vi "Test Coffee Shop Add Cashier.vi"(8 "error in (no error)":errorcluster, 11 "Coffee Shop Test In":refnum<class "Coffee Shop Test.lvclass">) -> (0 "error out":errorcluster, 3 "Coffee Shop Test Out":refnum<class "Coffee Shop Test.lvclass">)   [LabVIEW 2020, in "Coffee Shop Test.lvclass"]
uses:
  Coffee Shop Test.lvclass
  Coffee Shop/Coffee Shop.lvclass
  <vilib>/Asteme/Triarc Framework/Process/Process.lvclass
  <vilib>/Asteme/LUnit/Test Case.lvclass
  C:/Program Files (x86)/National Instruments/LabVIEW 2020/vi.lib/Asteme/Triarc Framework/Application/Application.lvclass
  C:/Program Files (x86)/National Instruments/LabVIEW 2020/vi.lib/Asteme/Triarc Framework/Process/Process.lvclass
  C:/Program Files (x86)/National Instruments/LabVIEW 2020/vi.lib/Asteme/Triarc Framework/Base/Base.lvclass
  C:/Program Files (x86)/National Instruments/LabVIEW 2020/vi.lib/Asteme/Triarc Framework/Error Handler Interface/Error Handler Interface.lvclass
  C:/Program Files (x86)/National Instruments/LabVIEW 2020/vi.lib/Asteme/Triarc Framework/Logging/Logging.lvclass
  C:/Users/anton/Documents/GitHub/Triarc-Examples/Coffee Shop/Coffee Shop/Coffee Shop.lvclass
  <vilib>/Asteme/Triarc Framework/Application/Application.lvclass
  C:/Program Files (x86)/National Instruments/LabVIEW 2020/vi.lib/Asteme/Triarc Framework Test Suite/Application Test/Application Test.lvclass
  C:/Program Files (x86)/National Instruments/LabVIEW 2020/vi.lib/Asteme/Triarc Framework Test Suite/Process Test/Process Test.lvclass
  C:/Program Files (x86)/National Instruments/LabVIEW 2020/vi.lib/Asteme/Triarc Framework Test Suite/Base Class Test/Base Test.lvclass
  C:/Program Files (x86)/National Instruments/LabVIEW 2020/vi.lib/Asteme/LUnit/Test Case.lvclass
  C:/Users/anton/Documents/GitHub/Triarc-Examples/Coffee Shop/Coffee Shop Test/Coffee Shop Test.lvclass
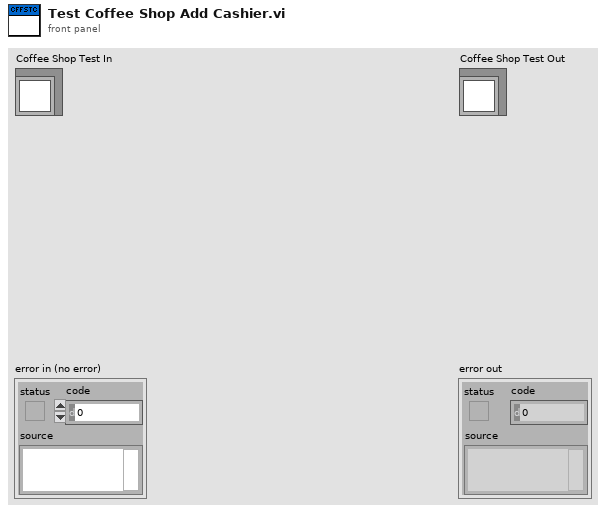
[diagram p1: front panel]
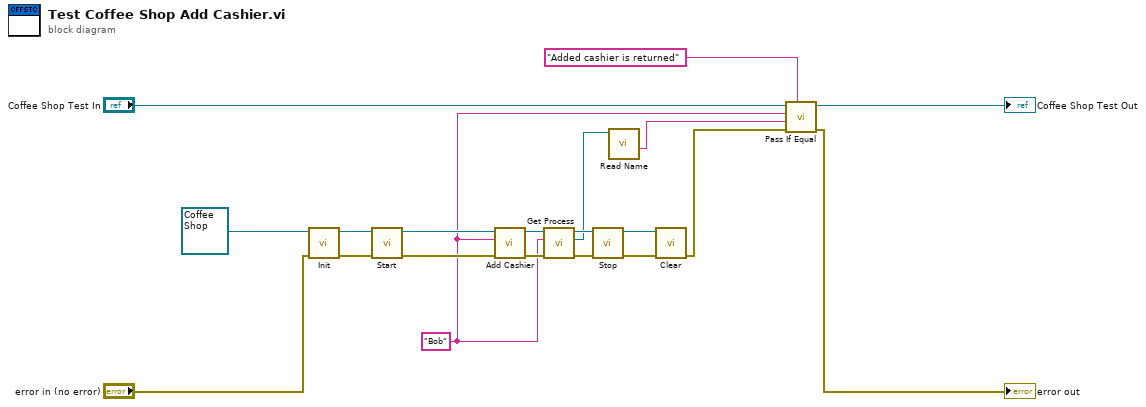
[diagram p0: block diagram]
diagram:
  w3 = "Bob" ("Name")
  n1 = call-dynamic "Init.vi"("error in (no error)"="error in (no error)", "Process In"=refnum<class "Coffee Shop.lvclass"> refnum ("Coffee Shop.lvclass")) -> ("error out"=w18:errorcluster, "Process Out"=w19:refnum<class "Coffee Shop.lvclass">)  [unwired: 8 in]
  n2 = call <vilib>:"Start.vi"("error in (no error)"=w18, "Process In"=w19) -> ("error out"=w13:errorcluster, "Process Out"=w12:refnum<class "Coffee Shop.lvclass">)  [unwired: 8 in]
  n3 = call "Add Cashier.vi"("error in (no error)"=w13, "Name"=w3, "Coffee Shop in"=w12) -> ("error out"=w14:errorcluster, "Coffee Shop out"=w5:refnum<class "Coffee Shop.lvclass">)  [unwired: 7 in]
  n4 = call <vilib>:"Get Process.vi"("error in (no error)"=w14, "Process Name"=w3, "Rig In"=w5) -> ("error out"=w6:errorcluster, "App Process"=w2:refnum<class "Process.lvclass">, "Rig Out"=w4:refnum<class "Coffee Shop.lvclass">)  [unwired: 6 in]
  n5 = call <vilib>:"Stop.vi"("error in (no error)"=w6, "Process In"=w4) -> ("error out"=w16:errorcluster, "Process Out"=w17:refnum<class "Coffee Shop.lvclass">)  [unwired: 7 in, 1 out]
  n6 = call-dynamic "Read Name.vi"("Process In"=w2) -> ("Name"=w1:string)  [unwired: 7 in, 3 out]
  n7 = call-dynamic "Clear.vi"("error in (no error)"=w16, "Application In"=w17) -> ("error out"=w9:errorcluster)  [unwired: 9 in]
  n8 = call <vilib>:"Pass If Equal.vi"("Description"="Added cashier is returned", "error in (no error)"=w9, "Actual"=w1, "Expected"=w3, "Test Case In"="Coffee Shop Test In") -> ("error out"=→"error out":errorcluster, "Test Case Out"=→"Coffee Shop Test Out":refnum<class "Coffee Shop Test.lvclass">)  [unwired: 5 in]
